vi "Write Data.vi"(8 "error in (no error)":errorcluster, 9 "Publication Time":timestamp, 10 "Value":variant, 11 "BooleanTextBinding In":refnum<class "BooleanTextBinding.lvclass">) -> (0 "error out":errorcluster, 3 "BooleanTextBinding Out":refnum<class "BooleanTextBinding.lvclass">)   [LabVIEW 2017, in "BooleanTextBinding.lvclass"]
doc: "<License>\nCopyright © 2017 Composed Systems, LLC | All rights reserved\nwww.composed.io\n\nAuthor: Ethan Stern <ethan.stern@composed.io>\n\nThis software is provided \"AS IS\" WITHOUT WARRANTIES, either express or implied, AND IS FOR EDUCATIONAL PURPOSES ONLY.\n</License>"
uses:
  <vilib>/gpm_packages/@cs/transport/Source/Concrete/BooleanTextBinding/BooleanTextBinding.lvclass
  <vilib>/gpm_packages/@cs/transport/Source/Concrete/BooleanTextBinding/BooleanTextBinding.lvclass/BooleanTextBinding.ctl
  <vilib>/Utility/error.llb/Error Cluster From Error Code.vi
  <vilib>/ErrorRing/Error Ring.xnode
  <vilib>/Utility/Data Type/NI_Data Type.lvlib
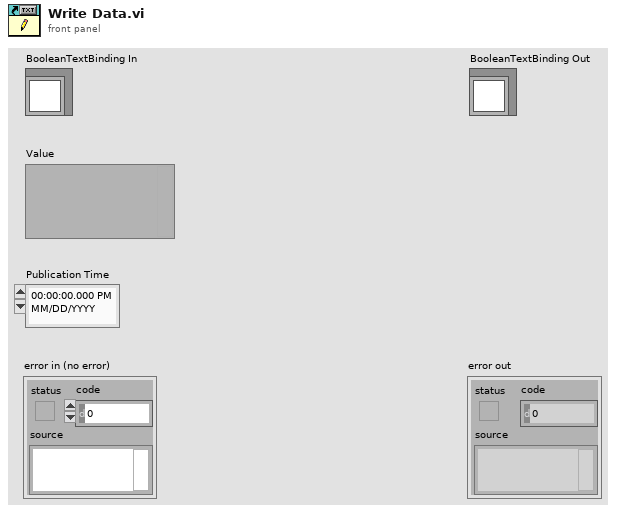
[diagram p1: front panel]
types:
  T1 = typedef "NI_Data Type.lvlib/Data Type.ctl" = enum8{"Invalid Type", "Void", "I8", "I16", "I32", "I64", "U8", "U16", "U32", "U64", "Single Float", "Double Float", "Extended Float", "Single Complex", "Double Complex", "Extended Complex", "Enum U8", "Enum U16", "Enum U32", "Enum U64", "Single Float With Unit", "Double Float With Unit", "Extended Float With Unit", "Single Complex with Unit", "Double Complex with Unit", "Extended Complex with Unit", "Boolean", "String", "Path", "Picture", "Tag", "Array", "Cluster", "Variant", "LV Variant", "Waveform", "Timestamp", "Digital Waveform", "Digital Data", "ExpressData", "Refnum", "External Data", "VI", "Poly VI", "LabVIEW Class Instance", "Fixed Point"}
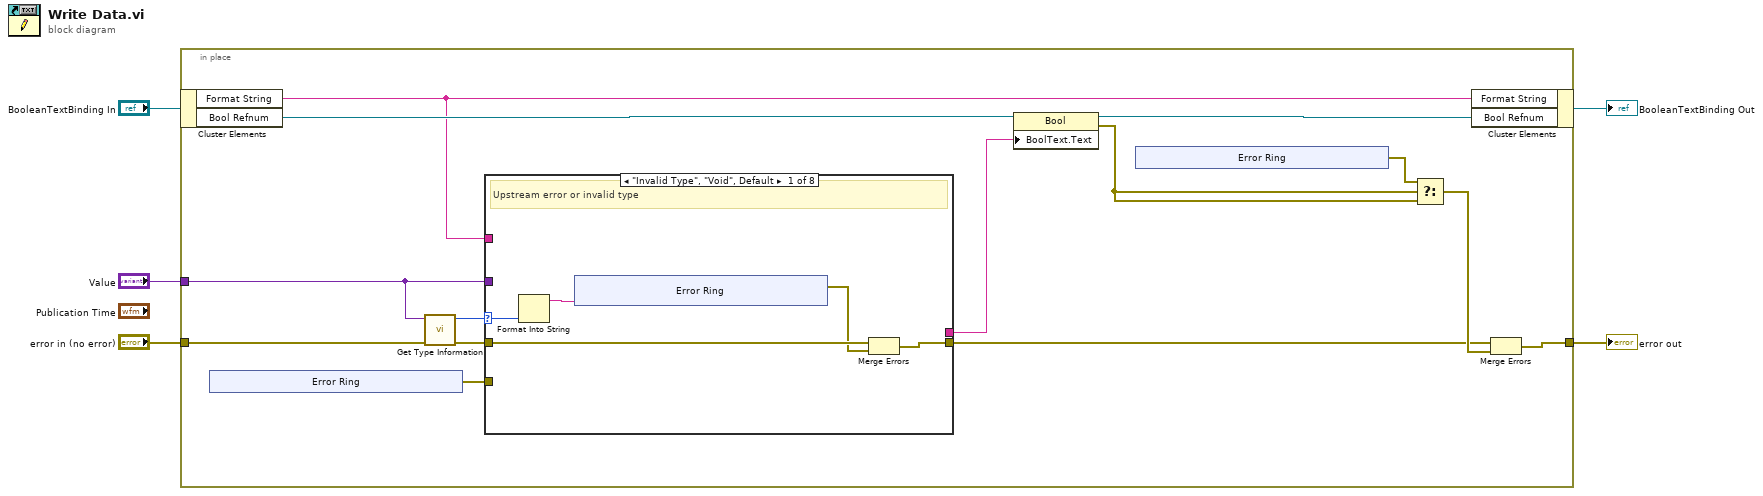
[diagram p0: block diagram]
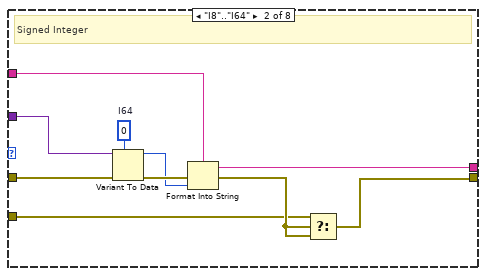
[diagram p2: hidden frame]
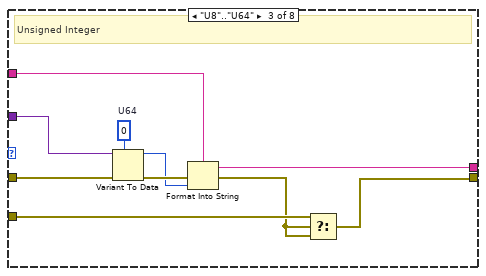
[diagram p3: hidden frame]
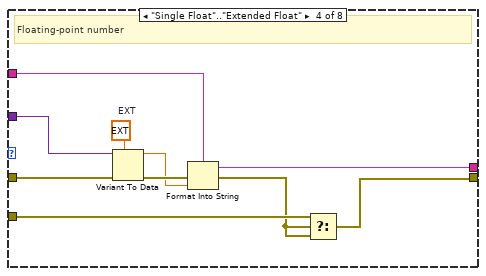
[diagram p4: hidden frame]
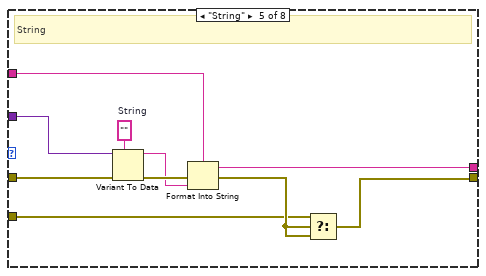
[diagram p5: hidden frame]
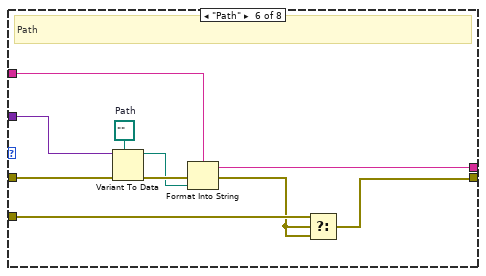
[diagram p6: hidden frame]
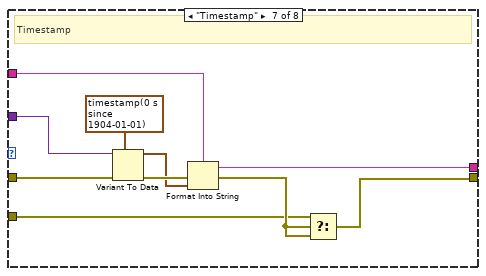
[diagram p7: hidden frame]
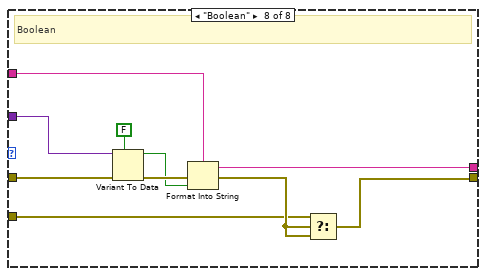
[diagram p8: hidden frame]
diagram:
  n1 = in-place {
    in-place-border: [w6] -> w5
    in-place-border: "Value" -> [w18]
    in-place-border: "error in (no error)" -> [w16]
    n2 = in-place-cluster #1("BooleanTextBinding In") -> ("Format String"=w12:string, "Bool Refnum"=w14:refnum<vi>)
    n3 = xnode "Error Ring"() -> ("error out"=w11:errorcluster)
    n4 = call <vilib>:"Get Type Information.vi"("error in (no error)"=w16, "Variant"=w18) -> ("error out"=w15:errorcluster, "Type"=w17:T1)  [unwired: 5 in, 3 out]
    n5 = case shown="\"Invalid Type\", \"Void\", Default" w17 {
      selector: w17 -> [w34 _ _ _ _ _ _ _]
      tunnel: w18 -> [_ w51 w61 w71 w81 w91 w101 w111]
      tunnel: w12 -> [_ w50 w60 w70 w80 w90 w100 w110]
      tunnel: [w32 w43 w52 w62 w72 w82 w93 w102] -> w7
      tunnel: [_ w48 w58 w68 w78 w88 w98 w108] -> w19
      tunnel: w15 -> [w31 w45 w55 w65 w75 w85 w95 w105]
      tunnel: w11 -> [_ w42 w54 w64 w73 w84 w92 w103]
      frame "Invalid Type", "Void", Default {
        # "Upstream error or invalid type"
        n6 = Format Into String(w34) -> (resulting string=w33:string)  [unwired: 3 in, 1 out]
        n7 = xnode "Error Ring"("parameter 0"=w33) -> ("error out"=w30:errorcluster)
        n8 = Merge Errors(w31, w30) -> (w32:errorcluster)
      }
      frame "I8".."I64" {
        w46 = i64 0  # I64
        # "Signed Integer"
        n9 = Variant To Data(error in=w45, type=w46, Variant=w51) -> (data=w47:i64, error out=w49:errorcluster)
        n10 = Format Into String(format string=w50, error in=w49, w47) -> (resulting string=w48:string, error out=w44:errorcluster)  [unwired: 1 in]
        n11 = Select(t=w42, s=w44, f=w44) -> (s? t:f=w43:errorcluster)
      }
      frame "U8".."U64" {
        w56 = u64 0  # U64
        # "Unsigned Integer"
        n12 = Variant To Data(error in=w55, type=w56, Variant=w61) -> (data=w57:u64, error out=w59:errorcluster)
        n13 = Format Into String(format string=w60, error in=w59, w57) -> (resulting string=w58:string, error out=w53:errorcluster)  [unwired: 1 in]
        n14 = Select(t=w54, s=w53, f=w53) -> (s? t:f=w52:errorcluster)
      }
      frame "Single Float".."Extended Float" {
        w66 = ext 0.0  # EXT
        # "Floating-point number"
        n15 = Variant To Data(error in=w65, type=w66, Variant=w71) -> (data=w67:ext, error out=w69:errorcluster)
        n16 = Format Into String(format string=w70, error in=w69, w67) -> (resulting string=w68:string, error out=w63:errorcluster)  [unwired: 1 in]
        n17 = Select(t=w64, s=w63, f=w63) -> (s? t:f=w62:errorcluster)
      }
      frame "String" {
        w76 = ""  # String
        # "String"
        n18 = Variant To Data(error in=w75, type=w76, Variant=w81) -> (data=w77:string, error out=w79:errorcluster)
        n19 = Format Into String(format string=w80, error in=w79, w77) -> (resulting string=w78:string, error out=w74:errorcluster)  [unwired: 1 in]
        n20 = Select(t=w73, s=w74, f=w74) -> (s? t:f=w72:errorcluster)
      }
      frame "Path" {
        w86 = path ""  # Path
        # "Path"
        n21 = Variant To Data(error in=w85, type=w86, Variant=w91) -> (data=w87:path, error out=w89:errorcluster)
        n22 = Format Into String(format string=w90, error in=w89, w87) -> (resulting string=w88:string, error out=w83:errorcluster)  [unwired: 1 in]
        n23 = Select(t=w84, s=w83, f=w83) -> (s? t:f=w82:errorcluster)
      }
      frame "Timestamp" {
        # "Timestamp"
        n24 = Variant To Data(error in=w95, type=timestamp(0 s since 1904-01-01) ("Timestamp"), Variant=w101) -> (data=w97:timestamp, error out=w99:errorcluster)
        n25 = Format Into String(format string=w100, error in=w99, w97) -> (resulting string=w98:string, error out=w94:errorcluster)  [unwired: 1 in]
        n26 = Select(t=w92, s=w94, f=w94) -> (s? t:f=w93:errorcluster)
      }
      frame "Boolean" {
        # "Boolean"
        n27 = Variant To Data(error in=w105, type=FALSE, Variant=w111) -> (data=w107:bool, error out=w109:errorcluster)
        n28 = Format Into String(format string=w110, error in=w109, w107) -> (resulting string=w108:string, error out=w104:errorcluster)  [unwired: 1 in]
        n29 = Select(t=w103, s=w104, f=w104) -> (s? t:f=w102:errorcluster)
      }
    }
    n30 = property class="Bool"(reference=w14, "BoolText.Text"=w19) -> (reference out=w13:refnum<vi>, error out=w10:errorcluster)  [unwired: 1 in]
    n31 = xnode "Error Ring"() -> ("error out"=w9:errorcluster)
    n32 = Select(t=w9, s=w10, f=w10) -> (s? t:f=w8:errorcluster)
    n33 = in-place-cluster #1("Format String"=w12, "Bool Refnum"=w13) -> (→"BooleanTextBinding Out":refnum<class "BooleanTextBinding.lvclass">)
    n34 = Merge Errors(w7, w8) -> (w6:errorcluster)
  }
  "error out" <- w5
